vi "Get Stop Event.vi"(8 "error in (no error)":errorcluster, 11 "User Interface Events in":refnum<class "User Interface Events.lvclass">) -> (0 "error out":errorcluster, 2 "stop event":refnum<user-event>, 3 "User Interface Events out":refnum<class "User Interface Events.lvclass">)   [LabVIEW 2017, in "DSF Core.lvlib" / "User Interface Events.lvclass"]
uses:
  User Interface Events.lvclass
  User Interface Events.lvclass/User Interface Events.ctl
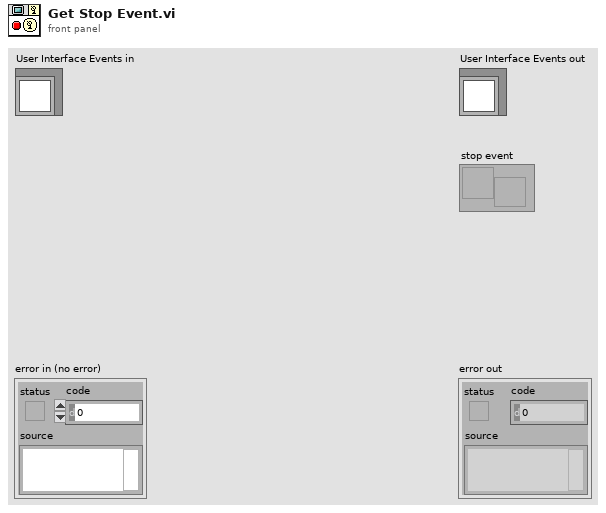
[diagram p1: front panel]
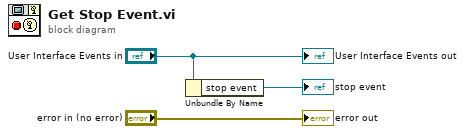
[diagram p0: block diagram]
diagram:
  n1 = Unbundle By Name("User Interface Events in") -> ("stop event"=→"stop event":refnum<user-event>)
  "error out" <- "error in (no error)"
  "User Interface Events out" <- "User Interface Events in"
